vi "Function 0 WhiteBox Tester.vi"() -> ()   [LabVIEW 2023]
uses:
  Drivers/Resideo Gas Valve/Type Definitions/Vesta Info.ctl
  Drivers/Resideo Gas Valve/Type Definitions/Temperature Control.ctl
  controls/Burner Duty Cycle.ctl
  controls/Timer Application Cluster.ctl
  controls/UI Data.ctl
panel:
  in  "Burner":bool
  in  "Main Burner Flag":bool
  in  "Differential Actual (F)":dbl
  in  "Setpoint Location (F)":dbl
  in  "Setpoint Actual (F)":dbl
  out "Data Cluster Out":T1={"Vesta Data Output"={"Temp_W_Raw_U"=0, "Temp_W_Raw_L"=0, "Temperature Water (F)"=0.0, "Temperature Water Compensated (F)"=0.0, "Temperature Ambient (F)"=0.0, "Setpoint Location (F)"=0.0, "Heat Request"="", "Fault Ram"="", "PWM DCDC Value"=0, "Pilot Voltage (mV)"=0.0, "Setpoint Actual (F)"=0.0, "Differential Actual (F)"=0.0, "Setpoint User (F)"=0.0, "Differential User (F)"=0.0, "Termperature FIltered -TCO (F)"=0.0, "Temp_C_Raw_1 - Sensor Voltage"="", "Temp_C_Raw_2 - Sensor Voltage"="", "Chamber Sensor Temperature (F)"=0.0, "LDO Base Temperature (F)"=0.0, "LDO Timer (sec)"=0, "Disabled (0)"=FALSE, "Warming (1)"=FALSE, "Heating (2)"=FALSE, "Cooling Data Write (3)"=FALSE, "Cooling (4)"=FALSE, "Data Read (5)"=FALSE, "N/A"=FALSE, "Temperature Trip (7)"=FALSE, "Burner"=FALSE}, "VestaTemperature"={"Water Heater Temp (°F)"=135, "Differential  (°F)"=10.0}, "Timer Application Data"={"Duty Cycle"={"Burner ON Time (Seconds)"=60.0, "Burner OFF Time (Seconds)"=60.0, "Main Burner Flag"=FALSE, "Burner Power Mode"=0}}, "Data Array"=[]} {"VestaTemperature"."Water Heater Temp (°F)" min=32 max=203}
  in  "Data Cluster":T1={"Vesta Data Output"={"Temp_W_Raw_U"=0, "Temp_W_Raw_L"=0, "Temperature Water (F)"=0.0, "Temperature Water Compensated (F)"=0.0, "Temperature Ambient (F)"=0.0, "Setpoint Location (F)"=0.0, "Heat Request"="", "Fault Ram"="", "PWM DCDC Value"=0, "Pilot Voltage (mV)"=0.0, "Setpoint Actual (F)"=0.0, "Differential Actual (F)"=0.0, "Setpoint User (F)"=0.0, "Differential User (F)"=0.0, "Termperature FIltered -TCO (F)"=0.0, "Temp_C_Raw_1 - Sensor Voltage"="", "Temp_C_Raw_2 - Sensor Voltage"="", "Chamber Sensor Temperature (F)"=0.0, "LDO Base Temperature (F)"=0.0, "LDO Timer (sec)"=0, "Disabled (0)"=FALSE, "Warming (1)"=FALSE, "Heating (2)"=FALSE, "Cooling Data Write (3)"=FALSE, "Cooling (4)"=FALSE, "Data Read (5)"=FALSE, "N/A"=FALSE, "Temperature Trip (7)"=FALSE, "Burner"=FALSE}, "VestaTemperature"={"Water Heater Temp (°F)"=135, "Differential  (°F)"=10.0}, "Timer Application Data"={"Duty Cycle"={"Burner ON Time (Seconds)"=60.0, "Burner OFF Time (Seconds)"=60.0, "Main Burner Flag"=FALSE, "Burner Power Mode"=0}}, "Data Array"=[]} {"VestaTemperature"."Water Heater Temp (°F)" min=32 max=203}
  out "Send_Vesta_Message":u8
  out "Send_Timer_Message":u8
  in  "error in (no error)":errorcluster
  in  "stop":bool
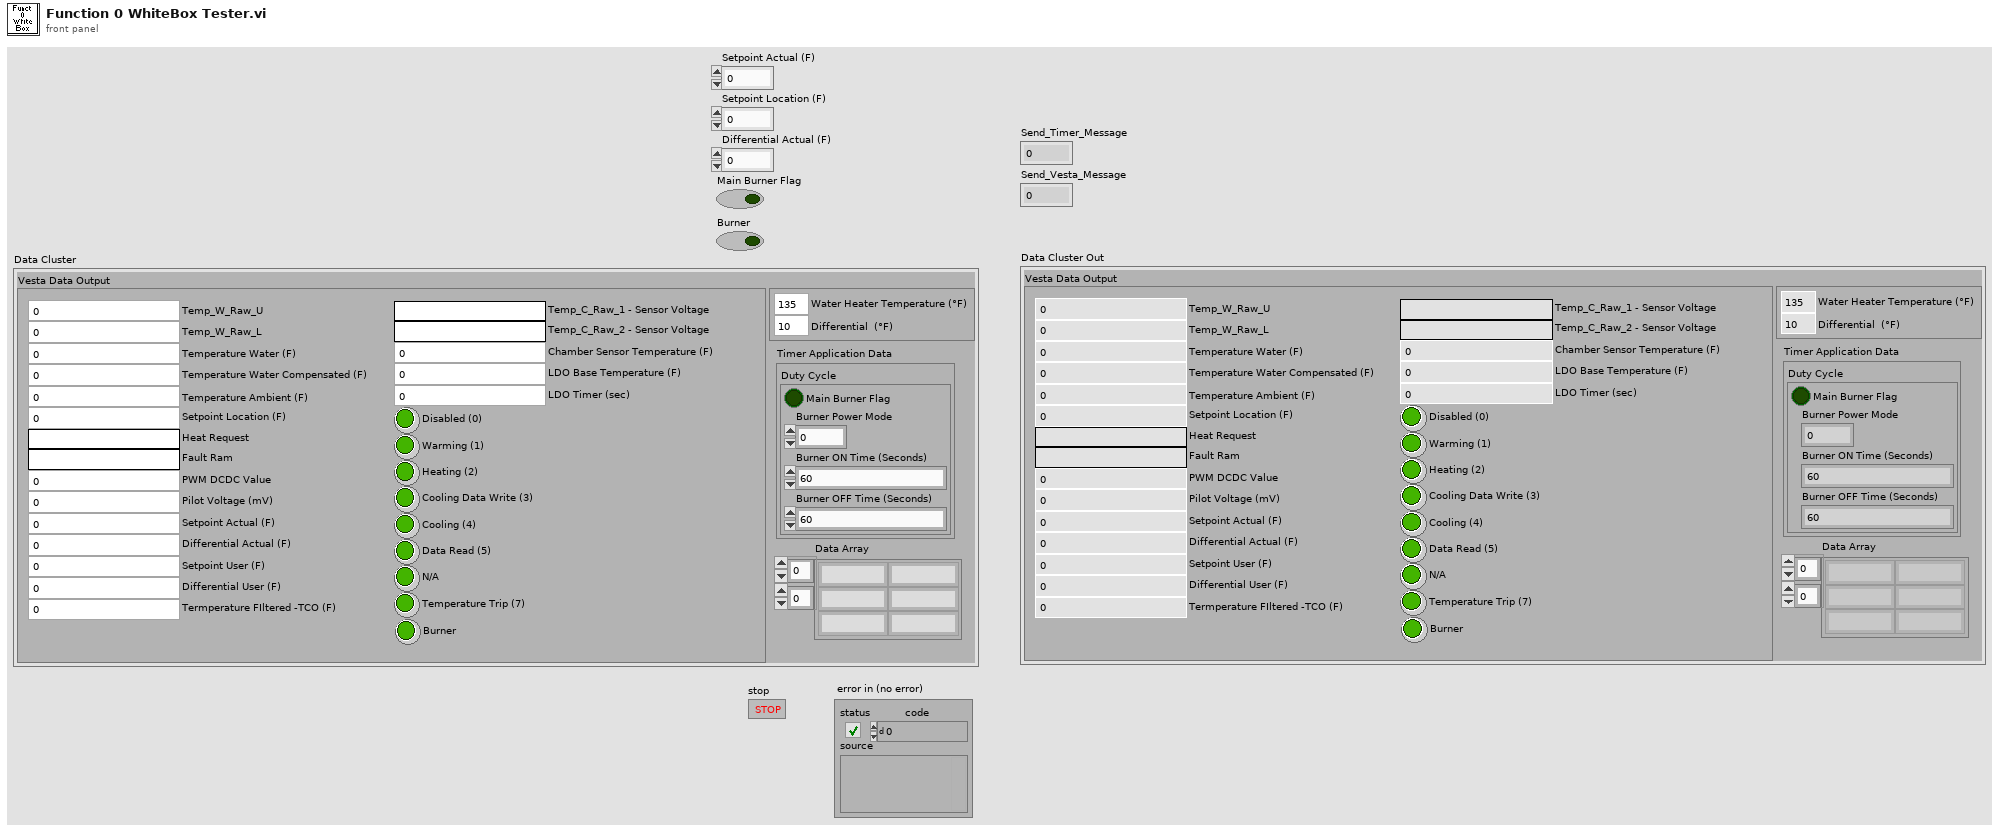
[diagram p1: front panel]
types:
  T1 = typedef "UI Data.ctl" = cluster{"Vesta Data Output":T2, "VestaTemperature":T3, "Timer Application Data":T4, "Data Array":string[][]}
  T2 = typedef "Vesta Info.ctl" = cluster{"Temp_W_Raw_U":u16, "Temp_W_Raw_L":u16, "Temperature Water (F)":dbl, "Temperature Water Compensated (F)":dbl, "Temperature Ambient (F)":dbl, "Setpoint Location (F)":dbl, "Heat Request":string, "Fault Ram":string, "PWM DCDC Value":u16, "Pilot Voltage (mV)":dbl, "Setpoint Actual (F)":dbl, "Differential Actual (F)":dbl, "Setpoint User (F)":dbl, "Differential User (F)":dbl, "Termperature FIltered -TCO (F)":dbl, "Temp_C_Raw_1 - Sensor Voltage":string, "Temp_C_Raw_2 - Sensor Voltage":string, "Chamber Sensor Temperature (F)":dbl, "LDO Base Temperature (F)":dbl, "LDO Timer (sec)":i16, "Disabled (0)":bool, "Warming (1)":bool, "Heating (2)":bool, "Cooling Data Write (3)":bool, "Cooling (4)":bool, "Data Read (5)":bool, "N/A":bool, "Temperature Trip (7)":bool, "Burner":bool}
  T3 = typedef "Temperature Control.ctl" = cluster{"Water Heater Temp (°F)":u16, "Differential  (°F)":dbl}
  T4 = typedef "Timer Application Cluster.ctl" = cluster{"Duty Cycle":T5}
  T5 = typedef "Burner Duty Cycle.ctl" = cluster{"Burner ON Time (Seconds)":dbl, "Burner OFF Time (Seconds)":dbl, "Main Burner Flag":bool, "Burner Power Mode":u8}
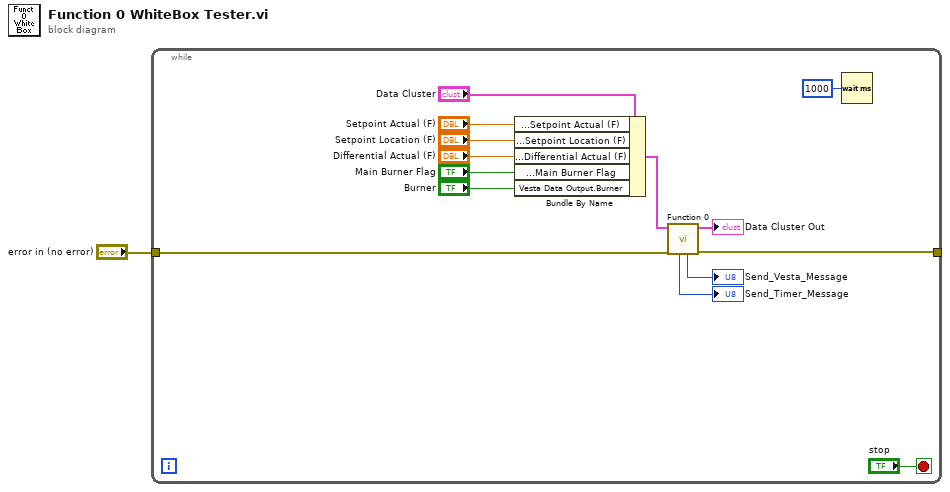
[diagram p0: block diagram]
diagram:
  n1 = while {
    tunnel: "error in (no error)" -> [w13]
    tunnel: [w12] -> _
    stop <- "stop" stop-if-true
    n2 = Bundle By Name(cluster="Data Cluster", "Vesta Data Output.Setpoint Actual (F)"="Setpoint Actual (F)", "Vesta Data Output.Setpoint Location (F)"="Setpoint Location (F)", "Vesta Data Output.Differential Actual (F)"="Differential Actual (F)", "Timer Application Data.Duty Cycle.Main Burner Flag"="Main Burner Flag", "Vesta Data Output.Burner"="Burner") -> (w7:T1)
    n3 = call "Function 0.vi"("error in (no error)"=w13, "Data Cluster"=w7) -> ("error out"=w12:errorcluster, "Data Cluster Out"=→"Data Cluster Out":T1, "Send_Vesta_Message"=→"Send_Vesta_Message":u8, "Send_Timer_Message"=→"Send_Timer_Message":u8)  [unwired: 6 in]
    n4 = Wait (ms)(milliseconds to wait=u32 1000) -> ()  [unwired: 1 out]
  }
